vi "XY Multi Plot.vi"() -> ()   [LabVIEW 2023]
doc: "Uses the Plot Multi-XY VI to draw multiple plots in a single graph, where the graph is drawn in a picture indicator."
uses:
  <vilib>/picture/cartesn2.llb/XY Plot Type.ctl
panel:
  in  "XY Plot Cosmetics":T2(array[cluster])=[{"Color Box"=3381759, "plot type"=enum."connected squares", "baseline"=0.0}, {"Color Box"=6618880, "plot type"=enum."circles", "baseline"=0.0}, {"Color Box"=16768018, "plot type"=enum."connected circles", "baseline"=0.0}]
  out "2D Picture":picture
  # "Overview: Uses the Plot Multi-XY VI to draw a multiple plots in a single 2D Picture Control.\nInstructions:\n1. Run the VI.\n2. Modify the XY Plot Cosmetics options to change the appearance of the graphs and run the VI again."
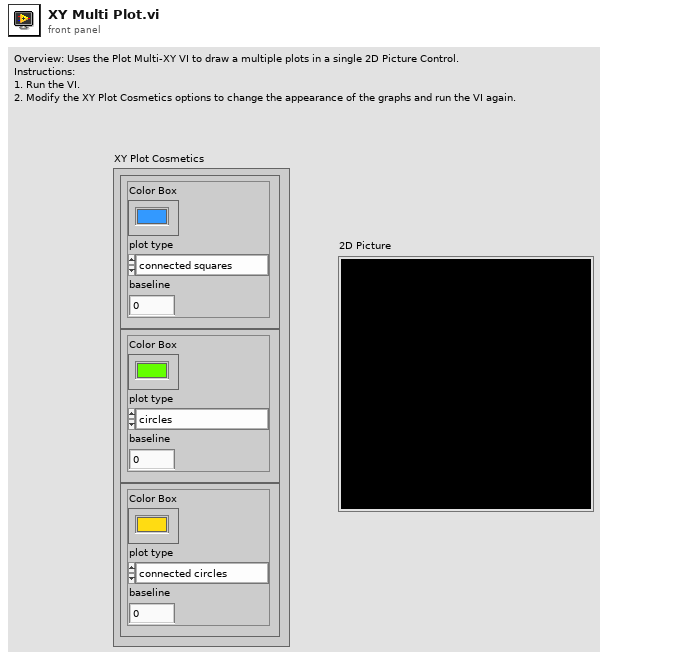
[diagram p1: front panel]
types:
  T1 = typedef "XY Plot Type.ctl" = enum16{"points", "squares", "circles", "connected points", "connected squares", "connected circles", "comb plot", "sized scatter plot", "sized-colored scatter plot", "min-max lines"}
  T2 = cluster{"Color Box":u32, "plot type":T1, "baseline":dbl}[]
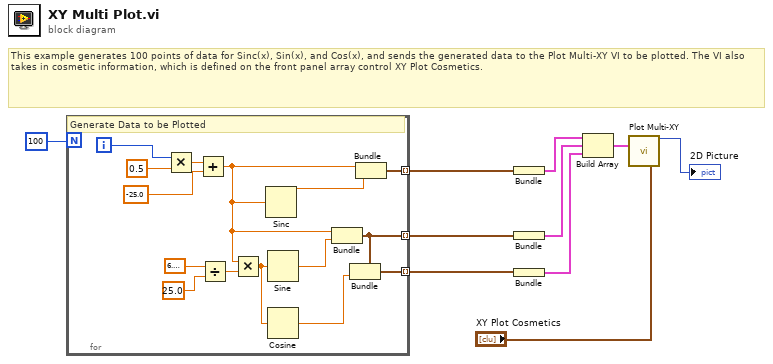
[diagram p0: block diagram]
diagram:
  # "This example generates 100 points of data for Sinc(x), Sin(x), and Cos(x), and sends the generated data to the Plot Multi-XY VI to be plotted. The VI also takes in cosmetic information, which is defined on the front panel array control XY Plot Cosmetics."
  n1 = for {
    N: 100 -> [_]
    tunnel: [w18] -> w8 mode=indexing
    tunnel: [w17] -> w7 mode=indexing
    tunnel: [w16] -> w6 mode=indexing
    i -> [w20]
    # "Generate Data to be Plotted"
    n2 = Multiply(x=w20, y=0.5) -> (x*y=w25:dbl)
    n3 = Add(x=w25, y=-25.0) -> (x+y=w14:dbl)
    n4 = Divide(x=6.283185307179586, y=25.0) -> (x/y=w23:dbl)
    n5 = Multiply(x=w14, y=w23) -> (x*y=w15:dbl)
    n6 = Sinc(1:w14) -> (0:w24:dbl)
    n7 = Sine(x=w15) -> (sin(x)=w21:dbl)
    n8 = Cosine(x=w15) -> (cos(x)=w19:dbl)
    n9 = Bundle(w14, w21) -> (w17:cluster{dbl, dbl})  [unwired: 1 in]
    n10 = Bundle(cluster=w17, w19) -> (w16:cluster{dbl, dbl})  [unwired: 1 in]
    n11 = Bundle(w14, w24) -> (w18:cluster{dbl, dbl})  [unwired: 1 in]
  }
  n12 = Bundle(w8) -> (w5:cluster{cluster{dbl, dbl}[]})  [unwired: 1 in]
  n13 = Bundle(w7) -> (w4:cluster{cluster{dbl, dbl}[]})  [unwired: 1 in]
  n14 = Bundle(w6) -> (w3:cluster{cluster{dbl, dbl}[]})  [unwired: 1 in]
  n15 = Build Array(w5, w4, w3) -> (w2:cluster{cluster{dbl, dbl}[]}[])
  n16 = call <vilib>:"Plot Multi-XY.vi"("data"=w2, "XY plot cosmetics"="XY Plot Cosmetics") -> ("new picture"=→"2D Picture":picture)  [unwired: 13 in]
